vi "niDTS WLAN INSTR RX Initiate.vi"(8 "error in (no error)":errorcluster, 9 "Result Instance":i32=1, 10 "Driver Instance":i32=1, 11 "niDTS WLAN INSTR RX in":refnum<class "niDTS WLAN INSTR RX.lvclass">) -> (0 "error out":errorcluster, 3 "niDTS WLAN INSTR RX out":refnum<class "niDTS WLAN INSTR RX.lvclass">)   [LabVIEW 2015, in "niDTS WLAN.lvlib" / "niDTS WLAN INSTR RX.lvclass"]
uses:
  niDTS WLAN INSTR RX.lvclass
  niDTS WLAN INSTR RX.lvclass/niDTS WLAN INSTR RX.ctl
  RiviInstDriver/niRfsgWlan/Objects/niRfsgWlan.lvclass
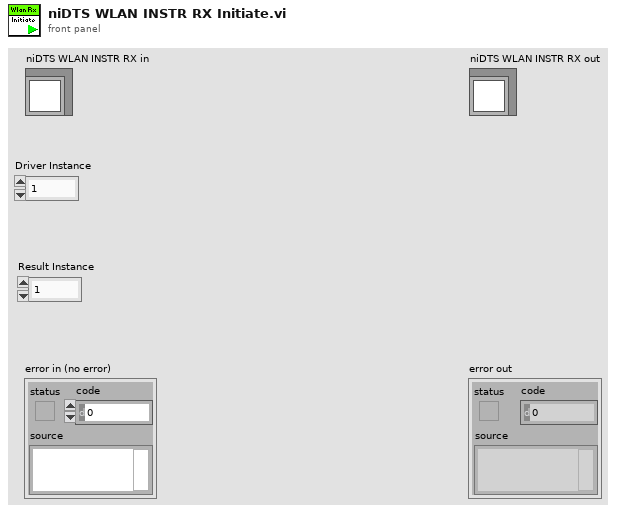
[diagram p1: front panel]
types:
  T1 = typedef "niRfsgWlan.lvclass/niRfsgWlan INC Handle.ctl" = refnum<data-value>
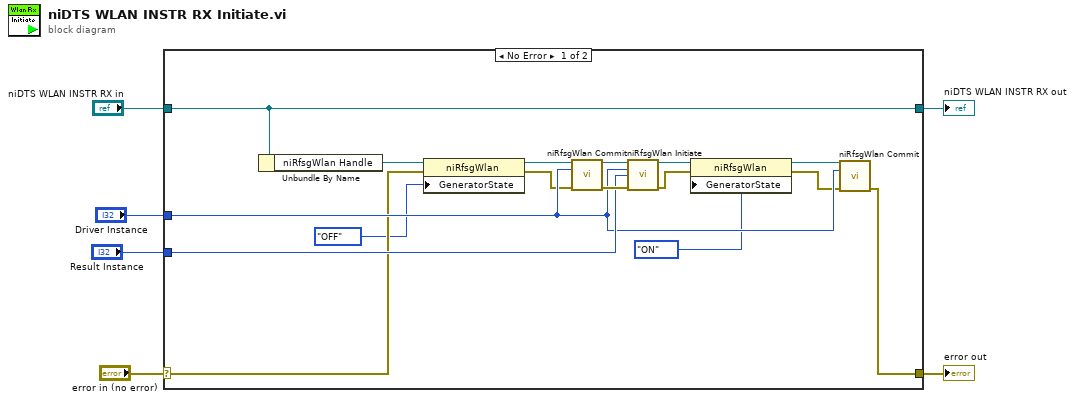
[diagram p0: block diagram]
diagram:
  n1 = case shown="No Error" "error in (no error)" {
    selector: "error in (no error)" -> [w10 w24]
    tunnel: [w13 w24] -> w5
    tunnel: [w20 w23] -> w3
    tunnel: "niDTS WLAN INSTR RX in" -> [w20 w23]
    tunnel: "Driver Instance" -> [w15 _]
    tunnel: "Result Instance" -> [w19 _]
    frame No Error {
      n2 = Unbundle By Name(w20) -> ("niRfsgWlan Handle"=w12:T1)
      n3 = property class="niRfsgWlan"(reference=w12, error in=w10, "GeneratorState"=enum16{"OFF", "PENDING", "ON"}."OFF" ("SOURce:RFSG:WLAN:GeneratorState")) -> (reference out=w11:T1, error out=w9:errorcluster)
      n4 = call "niRfsgWlan Commit.vi"("InstDriver Handle in"=w11, "Instance"=w15, "error in (no error)"=w9) -> ("InstDriver Handle out"=w21:T1, "error out"=w22:errorcluster)  [unwired: 11 in]
      n5 = call "niRfsgWlan Initiate.vi"("InstDriver Handle in"=w21, "Driver Instance"=w15, "Result Instance"=w19, "error in (no error)"=w22) -> ("InstDriver Handle out"=w18:T1, "error out"=w17:errorcluster)  [unwired: 10 in]
      n6 = property class="niRfsgWlan"(reference=w18, error in=w17, "GeneratorState"=enum16{"OFF", "PENDING", "ON"}."ON" ("SOURce:RFSG:WLAN:GeneratorState")) -> (reference out=w16:T1, error out=w14:errorcluster)
      n7 = call "niRfsgWlan Commit.vi"("InstDriver Handle in"=w16, "Instance"=w15, "error in (no error)"=w14) -> ("error out"=w13:errorcluster)  [unwired: 11 in, 1 out]
    }
    frame Error {
    }
  }
  "error out" <- w5
  "niDTS WLAN INSTR RX out" <- w3
